vi "Correct Non-Uniformity.vi"(8 "error in":errorcluster, 11 "ICorrect Non-Uniformity":refnum<class "ICorrect Non-Uniformity.lvclass">) -> (0 "error out":errorcluster, 3 "ICorrect Non-Uniformity out":refnum<class "ICorrect Non-Uniformity.lvclass">)   [LabVIEW 2024, in "ICorrect Non-Uniformity.lvclass"]
uses:
  ICorrect Non-Uniformity.lvclass
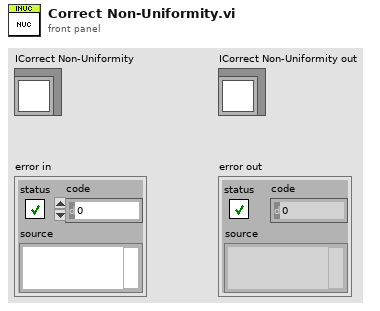
[diagram p1: front panel]
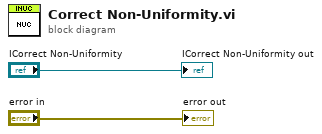
[diagram p0: block diagram]
diagram:
  "error out" <- "error in"
  "ICorrect Non-Uniformity out" <- "ICorrect Non-Uniformity"
